vi "AlarmChecks.vi"(9 "Settings":T1={"Name of test"="", "Date"=timestamp(0 s since 1904-01-01), "Location"="", "Template"="", "Soundcard"="", "resolution"=32, "Sampling rate"=48000, "Ch1 Gain "=25.0, "Ch2 Gain"=10.0, "Sample time (s)"=0.3, "Pre-trigger (s)"=0.01, "Hammer Threshold"=10.0, "Positions"=12, "Taps/Position"=5, "Set Names"="", "Freq resolution"=10.0, "Hammer cutoff"=0.0, "Mic cutoff"=0.0, "Double bounce "=0.0, "Hammer Cal"=10.0, "dB Offset"=0.0, "Accel Cal"=10.0, "Vibrometer Cal"=0.0, "Mic Cal"=0.0, "Output"=2, "Voltage Cal"=1.0, "Vibrometer Port"="ASRL27::INSTR", "Range"=4, "High Pass"=2, "Bandwidth"=4, "X Range"=[], "Y Range"=[], "dB Spread"=0.0, "Trigger"=0, "Ch_1"=25, "Ch_2"=25, "flip?"=FALSE, "60Hz"=FALSE, "Time offset"=0.0, "Piezo Cal"=1.0, "Default Notes"=""} {"Ch_2" min=1 step=1; "Ch_1" min=1 max=100 step=1; "Trigger" items=["Hammer (force)", "Self-tap", "Spacebar"]; "Bandwidth" items=["1 kHz"=1, "5 kHz"=5, "10 kHz"=10, "25 kHz"=25, "50 kHz"=50, "100 kHz"=100]; "High Pass" items=["Off", "13 Hz", "104 Hz"]; "Range" items=["10 mm/s"=1, "20 mm/s"=2, "50 mm/s"=5, "100 mm/s"=10, "200 mm/s"=20, "500 mm/s"=50, "1 m/s"=100, "2 m/s"=200]; "Output" items=["Accelerometer", "Speed (from acceleration)", "Microphone", "Vibrometer", "Piezo"]; "Voltage Cal" format="%#_13g"; "Ch2 Gain" format="%#_13g"; "Ch1 Gain" format="%#_13g"; "Double bounce" min=0.0; "Mic cutoff" min=0.0 format="%#_4g"; "Hammer cutoff" min=0.0 format="%#_4g"; "Freq resolution" min=0.0; "Pre-trigger (s)" format="%#_13g"; "Date" format="%<%H:%M\n%d/%m/%y>T"; "resolution" items=["16 bit"=16, "24 bit"=24, "32 bit"=32]; "Sampling rate" items=["22050 samp/s"=22050, "44100 samp/s"=44100, "48000 samp/s"=48000]}, 10 "Location":string, 11 "last tap":waveform(dbl)[](array[waveform])) -> (1 "Good point?":bool, 3 "Alarm":string)   [LabVIEW 2022 SP3]
uses:
  PreferencesControl.ctl
  Mic/Mic_Global.vi
panel:
  out "Waveform Graph":waveform(dbl)(graph)
  # "Hz"
  # "dB"
  # "dB"
  # "sec"
  # "sec"
  # "mV/Pa"
  # "mV/m/s2"
  # "mV/mm/s"
  # "V/N"
  # "sec"
  # "sec"
  # "mV/N"
  # "a.u."
  # "a.u."
  # "sec"
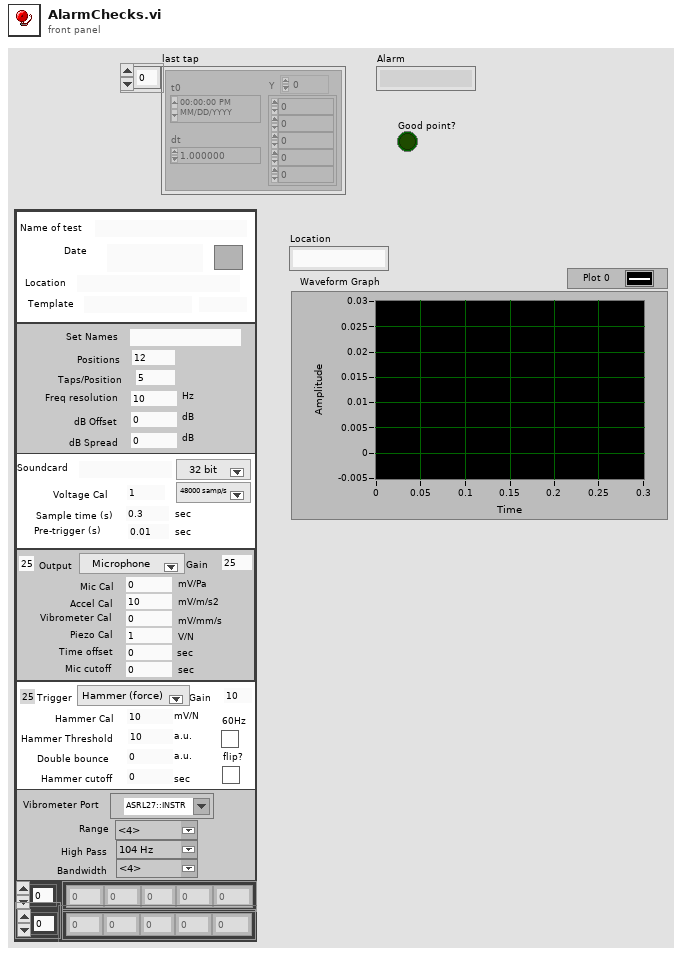
[diagram p1: front panel]
types:
  T1 = typedef "PreferencesControl.ctl" = cluster{"Name of test":string, "Date":timestamp, "Location":string, "Template":string, "Soundcard":string, "resolution":u16, "Sampling rate":u16, "Ch1 Gain ":dbl, "Ch2 Gain":dbl, "Sample time (s)":dbl, "Pre-trigger (s)":dbl, "Hammer Threshold":dbl, "Positions":i16, "Taps/Position":i16, "Set Names":string, "Freq resolution":dbl, "Hammer cutoff":dbl, "Mic cutoff":dbl, "Double bounce ":dbl, "Hammer Cal":dbl, "dB Offset":dbl, "Accel Cal":dbl, "Vibrometer Cal":dbl, "Mic Cal":dbl, "Output":u16, "Voltage Cal":dbl, "Vibrometer Port":refnum<visa-resource-name>, "Range":u16, "High Pass":u16, "Bandwidth":u16, "X Range":cluster{"Minimum":dbl, "Maximum":dbl, "Increment":dbl, "Minor Increment":dbl, "Start":dbl}[], "Y Range":cluster{"Minimum":dbl, "Maximum":dbl, "Increment":dbl, "Minor Increment":dbl, "Start":dbl}[], "dB Spread":dbl, "Trigger":u16, "Ch_1":u8, "Ch_2":u8, "flip?":bool, "60Hz":bool, "Time offset":dbl, "Piezo Cal":dbl, "Default Notes":string}
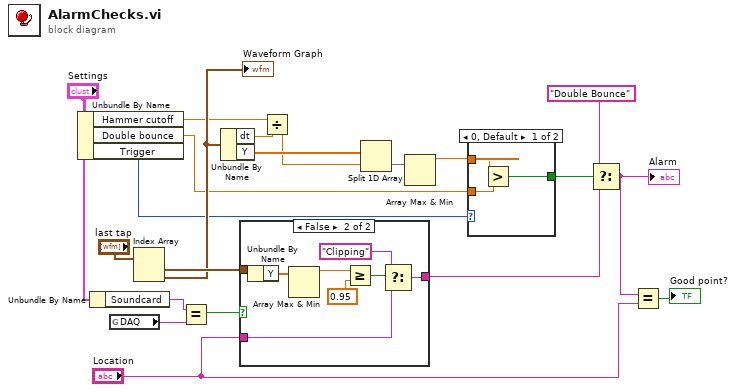
[diagram p0: block diagram]
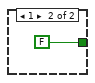
[diagram p3: hidden frame]
diagram:
  n1 = Unbundle By Name("Settings") -> ("Hammer cutoff"=w7:dbl, "Double bounce"=w6:dbl, "Trigger"=w5:u16)
  n2 = Unbundle By Name("Settings") -> ("Soundcard"=w2:string)
  n3 = global read "Mic_Global.vi" "DAQ"() -> (w3:string)
  n4 = Index Array(array="last tap") -> (element #1=w9:waveform(dbl), element #2=w8:waveform(dbl))  [unwired: 2 in]
  "Waveform Graph" <- w8
  n5 = Equal?(x=w2, y=w3) -> (x = y?=w1:bool)
  n6 = Unbundle By Name(w8) -> ("dt"=w15:dbl, "Y"=w17:dbl[])
  n7 = case shown="False" w1 {
    tunnel: [w22 w30] -> w19
    tunnel: "Location" -> [w22 w24]
    tunnel: w9 -> [_ w23]
    frame True {
    }
    frame False {
      n8 = Unbundle By Name(w23) -> ("Y"=w25:dbl[])
      n9 = Array Max & Min(array=w25) -> (max value=w26:dbl)  [unwired: 3 out]
      n10 = Greater Or Equal?(x=w26, y=0.95) -> (x >= y?=w28:bool)
      n11 = Select(t="Clipping" ("Alarm"), s=w28, f=w24) -> (s? t:f=w30:string)
    }
  }
  n12 = Divide(x=w7, y=w15) -> (x/y=w16:dbl)
  n13 = Split 1D Array(array=w17, index=w16) -> (second subarray=w10:dbl[])  [unwired: 1 out]
  n14 = Array Max & Min(array=w10) -> (max value=w14:dbl)  [unwired: 3 out]
  n15 = case shown="0, Default" w5 {
    tunnel: [w33 FALSE] -> w18
    tunnel: w14 -> [w32 _]
    tunnel: w6 -> [w31 _]
    frame 0, Default {
      n16 = Greater?(x=w32, y=w31) -> (0:w33:bool)
    }
    frame 1 {
    }
  }
  n17 = Select(t="Double Bounce" ("Alarm"), s=w18, f=w19) -> (s? t:f=w13:string)
  "Alarm" <- w13
  n18 = Equal?(x=w13, y="Location") -> (x = y?=→"Good point?":bool)
